vi "REPORT.Create Table.vi"(4 "delimiter (Tab)":string="\t", 5 "Secction":string, 6 "Row Headers":string[](array[string]), 7 "Column Headers":string[](array[string]), 8 "Text 2d":string[][](array[string]), 9 "Text In":string) -> (2 "output array":string[][](array[string]), 3 "Text Out":string)   [LabVIEW 2019]
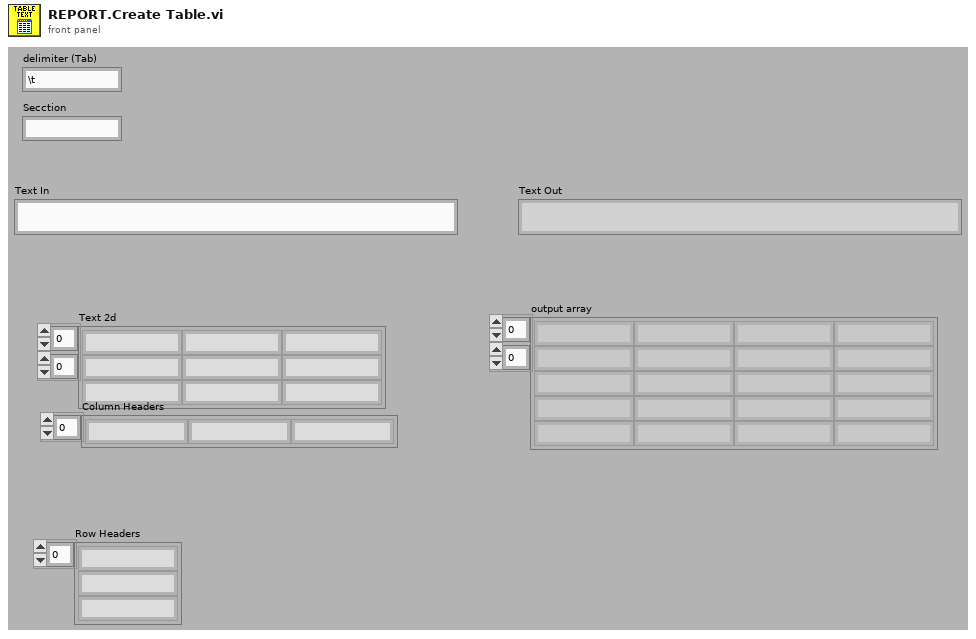
[diagram p1: front panel]
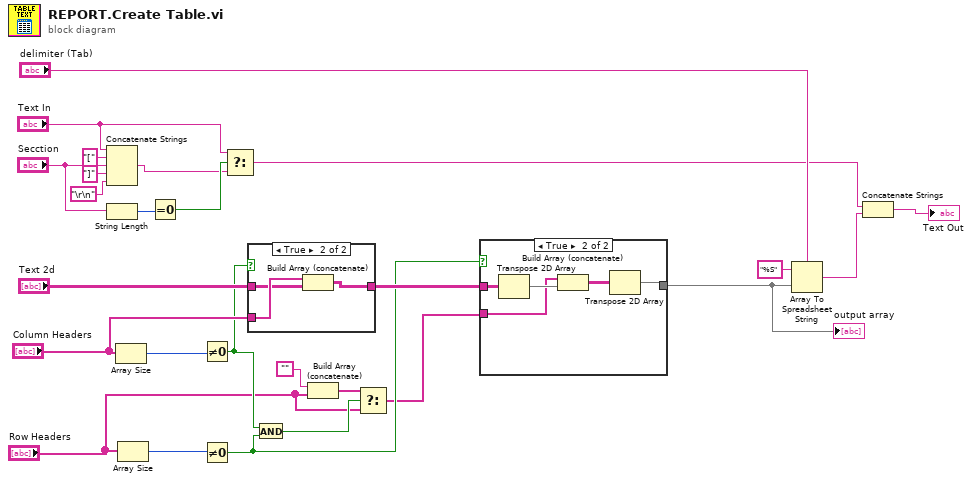
[diagram p0: block diagram]
diagram:
  n1 = Concatenate Strings("Text In", "[" ("string"), "Secction", "]" ("string"), "\r\n") -> (w3:string)
  n2 = String Length(string="Secction") -> (length=w6:i32)
  n3 = Array Size(array="Column Headers") -> (size(s)=w23:i32)
  n4 = Array Size(array="Row Headers") -> (size(s)=w22:i32)
  n5 = Equal To 0?(x=w6) -> (x = 0?=w5:bool)
  n6 = Not Equal To 0?(x=w23) -> (x != 0?=w18:bool)
  n7 = Not Equal To 0?(x=w22) -> (x != 0?=w17:bool)
  n8 = Select(t="Text In", s=w5, f=w3) -> (s? t:f=w2:string)
  n9 = case shown="True" w18 {
    tunnel: [w27 w28] -> w26
    tunnel: "Column Headers" -> [_ w30]
    tunnel: "Text 2d" -> [w27 w29]
    frame False {
    }
    frame True {
      n10 = Build Array (concatenate)(w30, w29) -> (w28:string[][])
    }
  }
  n11 = And(x=w18, y=w17) -> (x .and. y?=w15:bool)
  n12 = Build Array (concatenate)("", "Row Headers") -> (w14:string[])
  n13 = Select(t=w14, s=w15, f="Row Headers") -> (s? t:f=w12:string[])
  n14 = case shown="True" w17 {
    tunnel: w26 -> [w31 w36]
    tunnel: [w31 w32] -> w25
    tunnel: w12 -> [_ w34]
    frame False {
    }
    frame True {
      n15 = Transpose 2D Array(2D array=w36) -> (transposed array=w35:string[][])
      n16 = Build Array (concatenate)(w34, w35) -> (w33:string[][])
      n17 = Transpose 2D Array(2D array=w33) -> (transposed array=w32:string[][])
    }
  }
  "output array" <- w25
  n18 = Array To Spreadsheet String(delimiter (Tab)="delimiter (Tab)", array=w25, 3:"%S" ("format string")) -> (spreadsheet string=w11:string)
  n19 = Concatenate Strings(w2, w11) -> (→"Text Out":string)
